vi "Shift Registers Summation.vi"() -> ()   [LabVIEW 2019]
panel:
  out "sigma n":dbl
  in  "input n":sgl
  # "Challenge: \nSummation. Write a program that takes an input n and sums the integers from 1 to n."
  # "Try it: Enter a number in the \"input n\" box and hit Run."
  # "You will probably need:\nShift registers, for loops, numeric functions"
  # "Open the block diagram to see a possible solution."
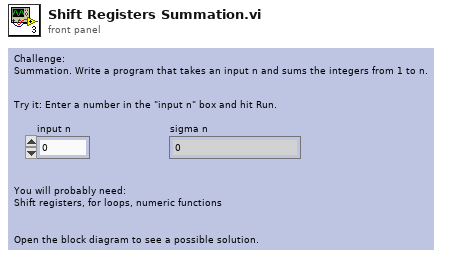
[diagram p1: front panel]
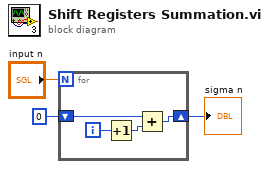
[diagram p0: block diagram]
diagram:
  n1 = for {
    N: "input n" -> [_]
    shift-right: [w4] -> w1
    shift-left: 0 -> [w5]
    i -> [w7]
    n2 = Increment(x=w7) -> (x+1=w6:i32)
    n3 = Add(x=w5, y=w6) -> (x+y=w4:i32)
  }
  "sigma n" <- w1
